vi "Stop Core.vi"(10 "final error code":i32, 11 "He Line in":refnum<class "He Line.lvclass">) -> (3 "He Line out":refnum<class "He Line.lvclass">)   [LabVIEW 2015, in "cRIO-Carbondioxide.lvlib" / "CO2-Actor.lvlib" / "He Line.lvclass"]
doc: "(<B>Filename</B>: Actor Framework.lvlib:Actor.lvclass:Stop Core.vi)\n\nDefines what the actor does before it stops. Use the <B>final error code</B> input to determine whether the actor shut down in response to an error.\n\nBy default, this method does nothing. A descendant class may override it to define behavior, such as shutting down any processes the actor initiated in its override of the Actor Core method."
uses:
  He Line.lvclass
  He Line.lvclass/He Line.ctl
  Valve/Valve.lvclass
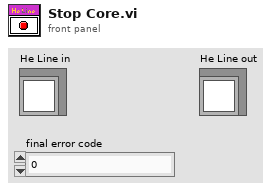
[diagram p1: front panel]
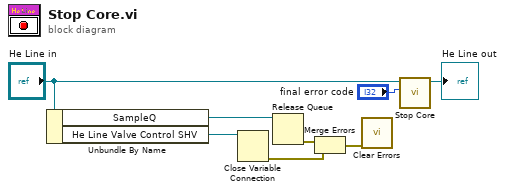
[diagram p0: block diagram]
diagram:
  n1 = Unbundle By Name("He Line in") -> ("SampleQ"=w5:refnum<queue>, "He Line Valve Control SHV"=w3:refnum<k21>)
  n2 = Close Variable Connection(11:w3) -> (0:w1:errorcluster)  [unwired: 1 in]
  n3 = Release Queue(queue=w5) -> (error out=w4:errorcluster)  [unwired: 2 in, 2 out]
  n4 = Merge Errors(w4, w1) -> (w2:errorcluster)
  n5 = call <vilib>:"Clear Errors.vi"("error in (no error)"=w2) -> ()  [unwired: 5 in, 2 out]
  n6 = call-parent "Stop Core.vi"("final error code"="final error code", "Valve in"="He Line in") -> ("Valve out"=→"He Line out":refnum<class "He Line.lvclass">)  [unwired: 9 in]
